vi "Factory Reset.vi"(8 "error in (no error)":errorcluster, 11 "EPU452 in":refnum<class "EPU452.lvclass">) -> (0 "error out":errorcluster, 2 "Response":string, 3 "EPU452 out":refnum<class "EPU452.lvclass">)   [LabVIEW 2018, in "EPU452.lvclass"]
uses:
  EPU452.lvclass
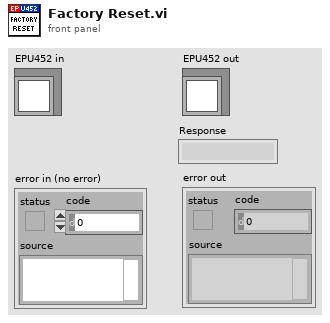
[diagram p1: front panel]
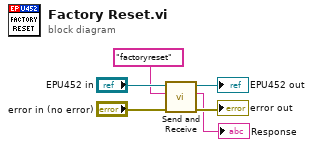
[diagram p0: block diagram]
diagram:
  n1 = call "Send and Receive.vi"("error in (no error)"="error in (no error)", "Command"="factoryreset", "EPU452 in"="EPU452 in") -> ("error out"=→"error out":errorcluster, "Response"=→"Response":string, "EPU452 out"=→"EPU452 out":refnum<class "EPU452.lvclass">)  [unwired: 6 in]
